vi "Remove Line From File.vi"(7 "Check Only? (f)":bool, 8 "Error In":errorcluster, 9 "Line":string="i2c-bcm2708", 10 "File Path":string="cat /etc/modules", 11 "Install LV Data":T1={"SSH Session"=refnum, "Status Log"="", "Detailed Log"="", "Credentials"={"Hostname or IP"="192.168.7.2", "Username"="root", "Password"=""}, "Target Info"={"OS Version"="", "CPU"="", "Systemd Version"="", "Internet Access"=FALSE, "Device Type"="", "LV Installed Ver"="", "LV Available Ver"="", "LV Upgrade Available"=FALSE, "Hostname"="", "NIC Info"=[]}, "Reboot Required?"=FALSE}) -> (0 "Error Out":errorcluster, 1 "Log":string, 2 "Line Previously Present?":bool, 3 "Install LV Data":T1={"SSH Session"=refnum, "Status Log"="", "Detailed Log"="", "Credentials"={"Hostname or IP"="192.168.7.2", "Username"="root", "Password"=""}, "Target Info"={"OS Version"="", "CPU"="", "Systemd Version"="", "Internet Access"=FALSE, "Device Type"="", "LV Installed Ver"="", "LV Available Ver"="", "LV Upgrade Available"=FALSE, "Hostname"="", "NIC Info"=[]}, "Reboot Required?"=FALSE})   [LabVIEW 2020, in "LMH-LINX.lvlib"]
uses:
  LMH-LINX.lvlib
  Install LV Data.ctl
  Target Info.ctl
  NIC Info.ctl
  NIC Mode.ctl
  <vilib>/regexp/Match Regular Expression.xnode
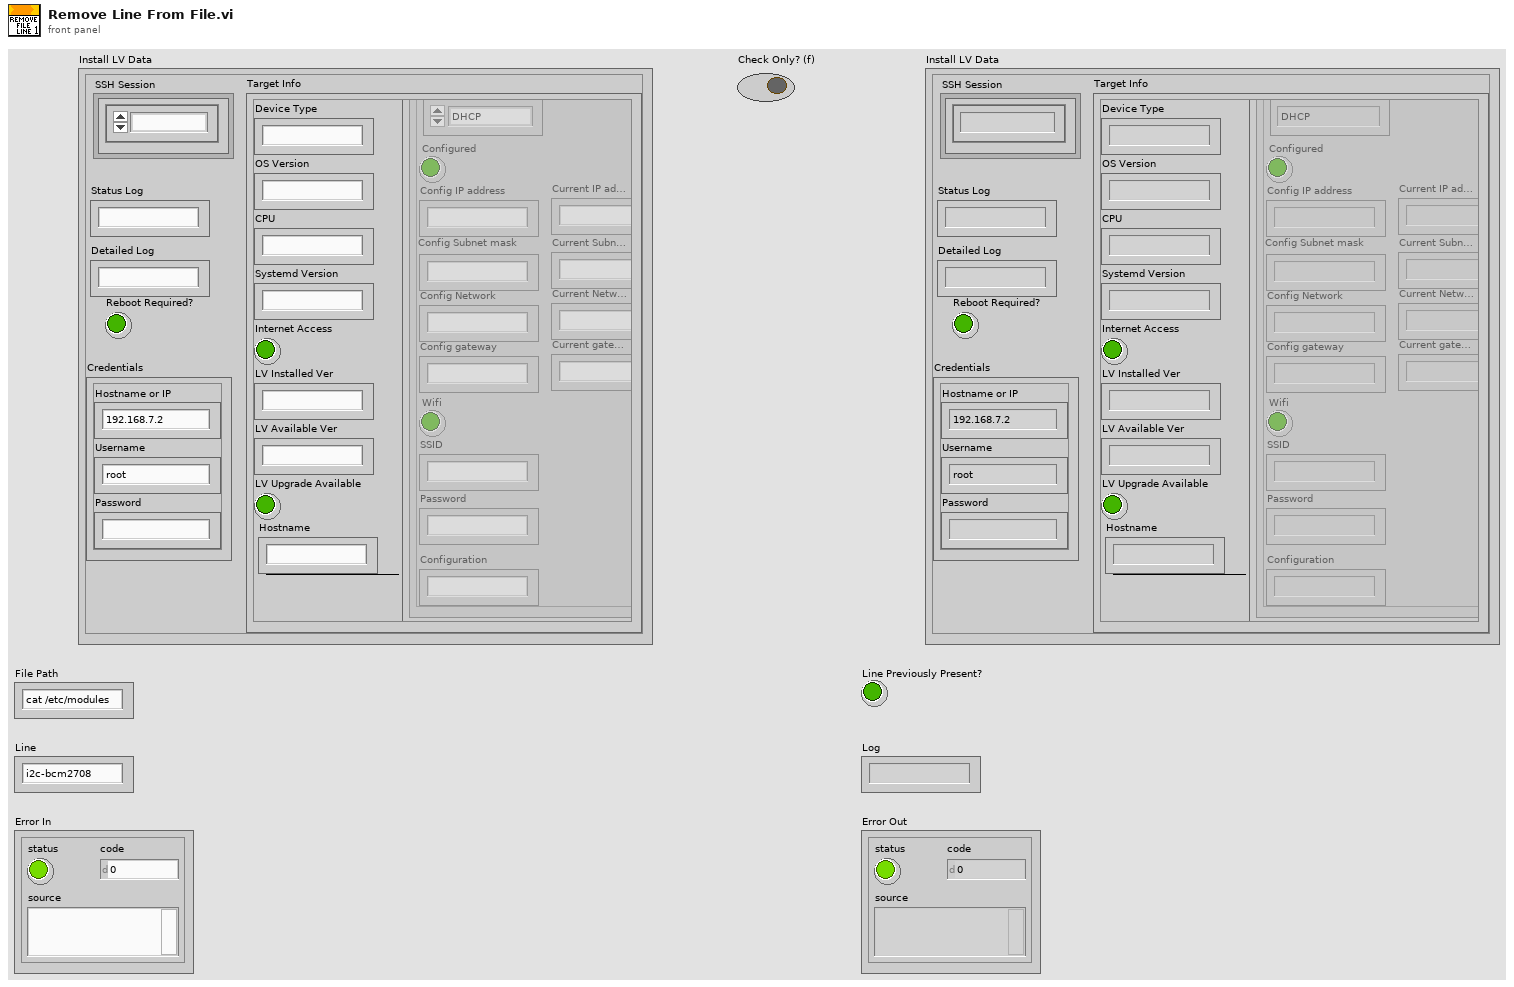
[diagram p1: front panel]
types:
  T1 = typedef "LMH-LINX.lvlib/Install LV Data.ctl" = cluster{"SSH Session":refnum<k1>, "Status Log":string, "Detailed Log":string, "Credentials":cluster{"Hostname or IP":string, "Username":string, "Password":string}, "Target Info":T2, "Reboot Required?":bool}
  T2 = typedef "LMH-LINX.lvlib/Target Info.ctl" = cluster{"OS Version":string, "CPU":string, "Systemd Version":string, "Internet Access":bool, "Device Type":string, "LV Installed Ver":string, "LV Available Ver":string, "LV Upgrade Available":bool, "Hostname":string, "NIC Info":T3[]}
  T3 = typedef "LMH-LINX.lvlib/NIC Info.ctl" = cluster{"Name":string, "NIC Mode":T4, "Configured":bool, "Config IP address":string, "Config Subnet mask":string, "Config Network":string, "Config gateway":string, "Wifi":bool, "SSID":string, "Password":string, "Configuration":string, "Current IP address":string, "Current Subnet mask":string, "Current gateway":string, "Current Network":string}
  T4 = typedef "LMH-LINX.lvlib/NIC Mode.ctl" = enum16{"DHCP", "Static", "Loopback"}
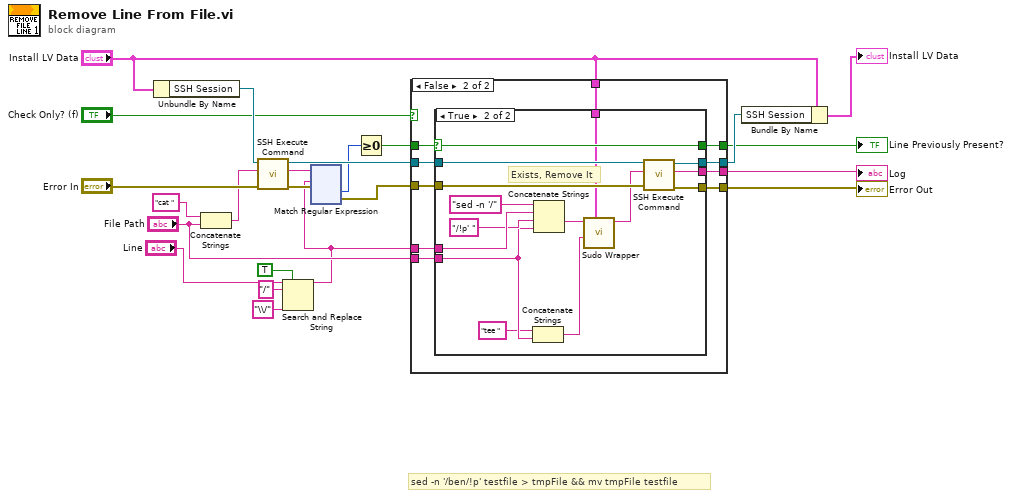
[diagram p0: block diagram]
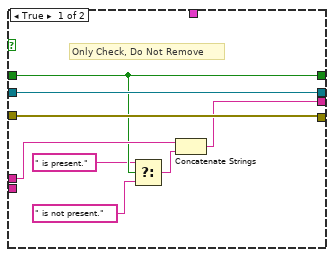
[diagram p2: hidden frame]
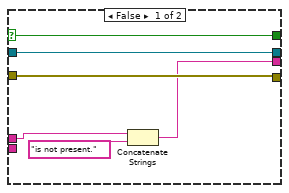
[diagram p3: hidden frame]
diagram:
  # "sed -n '/ben/!p' testfile > tmpFile && mv tmpFile testfile"
  n1 = Unbundle By Name("Install LV Data") -> ("SSH Session"=w22:refnum<k1>)
  n2 = Concatenate Strings("cat " ("string"), "File Path") -> (w13:string)
  n3 = call "SSH Execute Command.vi"("Error In"="Error In", "Command"=w13, "SSH Session"=w22) -> ("Error Out"=w19:errorcluster, "Std Out"=w15:string, "SSH Session"=w20:refnum<k1>)  [unwired: 6 in]
  n4 = Search and Replace String(replace all?=TRUE ("replace all? (F)"), input string="Line", search string="/", replace string="\\/" ("replace string (\"\")")) -> (result string=w2:string)  [unwired: 4 in, 3 out]
  n5 = xnode "Match Regular Expression"("input string"=w15, "regular expression"=w2, "error in"=w19) -> ("offset past match"=w17:i32, "error out"=w18:errorcluster)  [unwired: 3 in, 3 out]
  n6 = Greater Or Equal To 0?(x=w17) -> (x >= 0?=w16:bool)
  n7 = case shown="False" "Check Only? (f)" {
    tunnel: w20 -> [w31 w41]
    tunnel: w18 -> [w30 w40]
    tunnel: w16 -> [w27 w39]
    tunnel: w2 -> [w28 w38]
    tunnel: [w30 w37] -> w12
    tunnel: [w29 w36] -> w11
    tunnel: [w31 w35] -> w10
    tunnel: "File Path" -> [_ w34]
    tunnel: [w27 w33] -> w7
    tunnel: "Install LV Data" -> [_ w32]
    frame True {
      # "Only Check, Do Not Remove"
      n8 = Select(t=" is present.", s=w27, f=" is not present.") -> (s? t:f=w24:string)
      n9 = Concatenate Strings(w28, w24) -> (w29:string)
    }
    frame False {
      n10 = case shown="True" w39 {
        selector: w39 -> [w45 w58]
        tunnel: [w42 w54] -> w36
        tunnel: [w47 w62] -> w37
        tunnel: [w46 w61] -> w35
        tunnel: w41 -> [w46 w60]
        tunnel: w40 -> [w47 w59]
        tunnel: w38 -> [w44 w56]
        tunnel: w34 -> [_ w50]
        tunnel: [w45 w58] -> w33
        tunnel: w32 -> [_ w48]
        frame False {
          n11 = Concatenate Strings(w44, "is not present." ("string")) -> (w42:string)
        }
        frame True {
          # "Exists, Remove It"
          n12 = Concatenate Strings("tee ", w50) -> (w51:string)
          n13 = Concatenate Strings("sed -n '/", w56, "/!p' ", w50) -> (w53:string)
          n14 = call "Sudo Wrapper.vi"("Install LV Data"=w48, "comand string"=w51, "echo string"=w53) -> ("combined command string"=w52:string)  [unwired: 8 in]
          n15 = call "SSH Execute Command.vi"("Error In"=w59, "Command"=w52, "SSH Session"=w60) -> ("Error Out"=w62:errorcluster, "Std Out"=w54:string, "SSH Session"=w61:refnum<k1>)  [unwired: 6 in]
        }
      }
    }
  }
  "Log" <- w11
  "Error Out" <- w12
  "Line Previously Present?" <- w7
  n16 = Bundle By Name(cluster="Install LV Data", "SSH Session"=w10) -> (→"Install LV Data":T1)
